vi "SVL Get dB Reference (1 Ch).vi"(8 "error in (no error)":errorcluster, 11 "scaled signal [EU]":waveform(dbl)={"t0"=timestamp(0 s since 1904-01-01), "dt"=0.0, "Y"=[]}) -> (0 "error out":errorcluster, 2 "dB reference [EU]":dbl=nan format="%^.1e", 3 "scaled signal [EU]":waveform(dbl))   [LabVIEW 2017]
doc: "Returns the dB reference stored in the waveform attributes of the scaled signal input. The dB reference is set by the DAQ Assistant for Sound Pressure and Acceleration tasks, the SVL Scale Voltage to EU VI, and the SVL Set dB Reference VI. The dB reference is used for all downstream conversions to dB. Wire data to the <B>scaled signal [EU]</B> input to determine the polymorphic instance to use or manually select the instance."
uses:
  <vilib>/addons/_NISVFA/_Shared subVIs/Controls/svc_Channel Info.ctl
  <vilib>/addons/_NISVFA/_Shared subVIs/Controls/svc_Engineering Units Text Ring.ctl
  <vilib>/addons/_NISVFA/_Shared subVIs/Controls/svc_Weighting Filter Text Ring.ctl
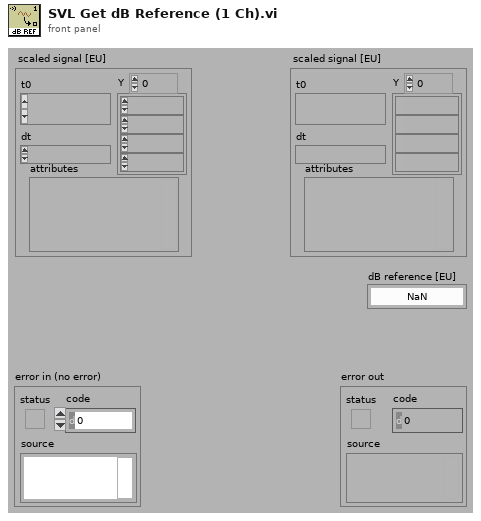
[diagram p1: front panel]
types:
  T1 = typedef "svc_Channel Info.ctl" = cluster{"sensor sensitivity":dbl, "engineering units":T2, "dB reference":dbl, "custom label":string, "weighting filter":T3, "pregain":dbl}
  T2 = typedef "svc_Engineering Units Text Ring.ctl" = u16
  T3 = typedef "svc_Weighting Filter Text Ring.ctl" = u16
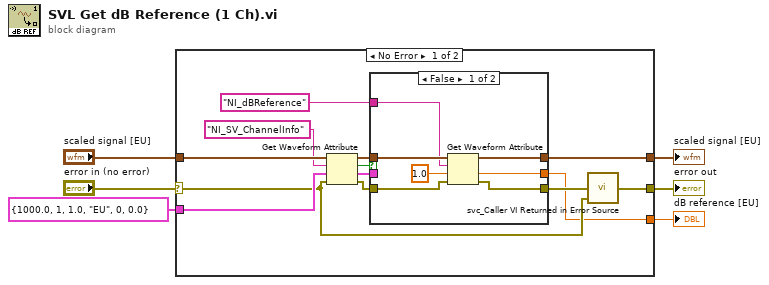
[diagram p0: block diagram]
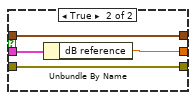
[diagram p2: hidden frame]
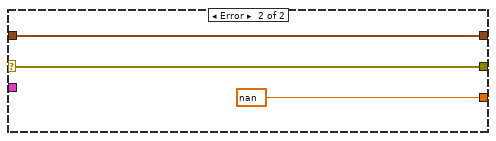
[diagram p3: hidden frame]
diagram:
  n1 = case shown="No Error" "error in (no error)" {
    selector: "error in (no error)" -> [w16 w33]
    tunnel: "scaled signal [EU]" -> [w19 w32]
    tunnel: [w17 w33] -> w5
    tunnel: [w8 w32] -> w4
    tunnel: T1 {"sensor sensitivity"=1000.0, "engineering units"=1, "dB reference"=1.0, "custom label"="EU", "weighting filter"=0, "pregain"=0.0} ("channel info") -> [w18 _]
    tunnel: [w7 nan ("dB reference [EU]")] -> w1
    frame No Error {
      n2 = Get Waveform Attribute(4:w16, 5:w18, 6:"NI_SV_ChannelInfo" ("name"), 7:w19) -> (0:w15:errorcluster, 1:w12:T1, 2:w11:bool, 3:w14:waveform(dbl))
      n3 = case shown="False" w11 {
        tunnel: w15 -> [w25 w30]
        tunnel: w14 -> [w24 w29]
        tunnel: w12 -> [_ w27]
        tunnel: "NI_dBReference" ("name") -> [w23 _]
        tunnel: [w21 w30] -> w9
        tunnel: [w20 w29] -> w8
        tunnel: [w22 w28] -> w7
        frame False {
          n4 = Get Waveform Attribute(4:w25, 5:1.0 ("dB reference [EU]"), 6:w23, 7:w24) -> (0:w21:errorcluster, 1:w22:dbl, 3:w20:waveform(dbl))  [unwired: 1 out]
        }
        frame True {
          n5 = Unbundle By Name(w27) -> ("dB reference"=w28:dbl)
        }
      }
      n6 = call <vilib>:"svc_Caller VI Returned in Error Source.vi"("warning input to caller"=w16, "error in (no error)"=w9) -> ("error out"=w17:errorcluster)  [unwired: 3 in]
    }
    frame Error {
    }
  }
  "scaled signal [EU]" <- w4
  "error out" <- w5
  "dB reference [EU]" <- w1
